vi "Actor Core.vi"(8 "error in":errorcluster, 11 "Nested in":refnum<class "Microscope Controller.lvclass">) -> (0 "error out":errorcluster, 3 "Actor out":refnum<class "Actor.lvclass">)   [LabVIEW 2020, in "Microscope.lvlib" / "Microscope Controller.lvlib" / "Microscope Controller.lvclass"]
doc: "(<B>Filename</B>: Actor Framework.lvlib:Actor.lvclass:Actor Core.vi)\n\nReceives messages to the actor, reacts to them, and initiates any error handling that may shut the actor down.\n\nDescendant classes may override this VI to append parallel tasks for the actor to complete while it handles messages. Overrides use the Call Parent Method node."
uses:
  Microscope Controller.lvclass
  C:/Program Files/National Instruments/LabVIEW 2020/vi.lib/ActorFramework/Actor/Actor.lvclass
  <vilib>/ActorFramework/Actor/Actor.lvclass
  <vilib>/ActorFramework/Actor/Actor.lvclass/Actor.ctl
  <vilib>/ActorFramework/Message Enqueuer/Message Enqueuer.lvclass/Message Enqueuer.ctl
  Microscope Controller.lvclass/Microscope Controller.ctl
  <vilib>/ActorFramework/Message Enqueuer/Init from Existing Queue.vi
  <vilib>/ActorFramework/Message Enqueuer/Enqueue.vi
  <vilib>/ActorFramework/Stop Msg/Stop Msg.lvclass
  C:/Program Files/National Instruments/LabVIEW 2020/vi.lib/ActorFramework/Message/Message.lvclass
  <vilib>/ActorFramework/Message Priority Queue/Priority Enqueue.vi
  <vilib>/ActorFramework/Message Enqueuer/Message Enqueuer.lvclass
panel:
  in  "Tab Control":T1(tab)
  out "SystemStatus":string
  # "430 Chemical and Biomedical Engineering Bldg.\nThe Pennsylvania State University"
  # "woh1@psu.edu"
  # "https://sites.psu.edu/hancocklab/"
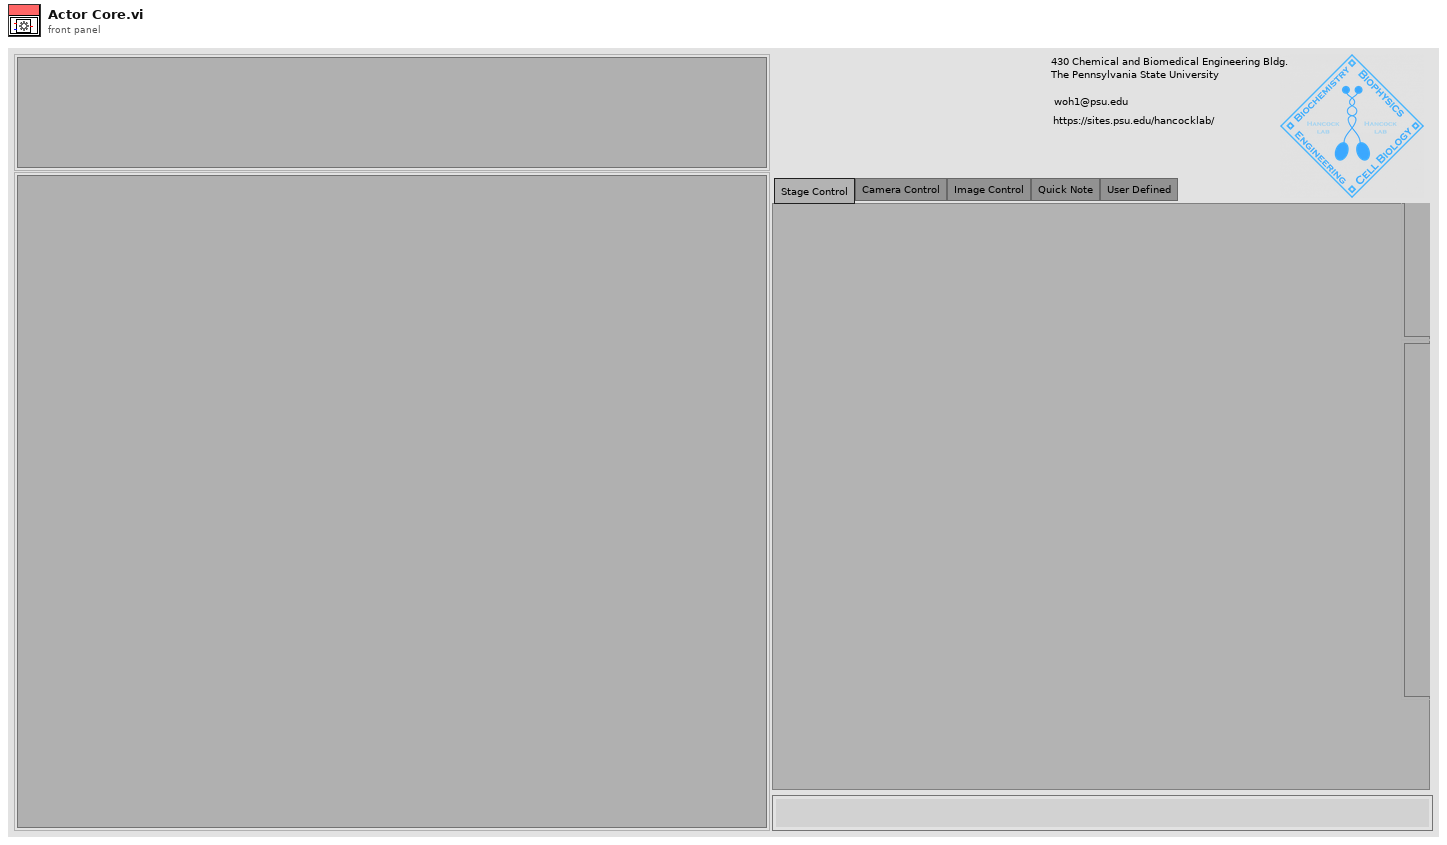
[diagram p1: front panel]
types:
  T1 = enum32{"Stage Control", "Camera Control", "Image Control", "Quick Note", "User Defined"}
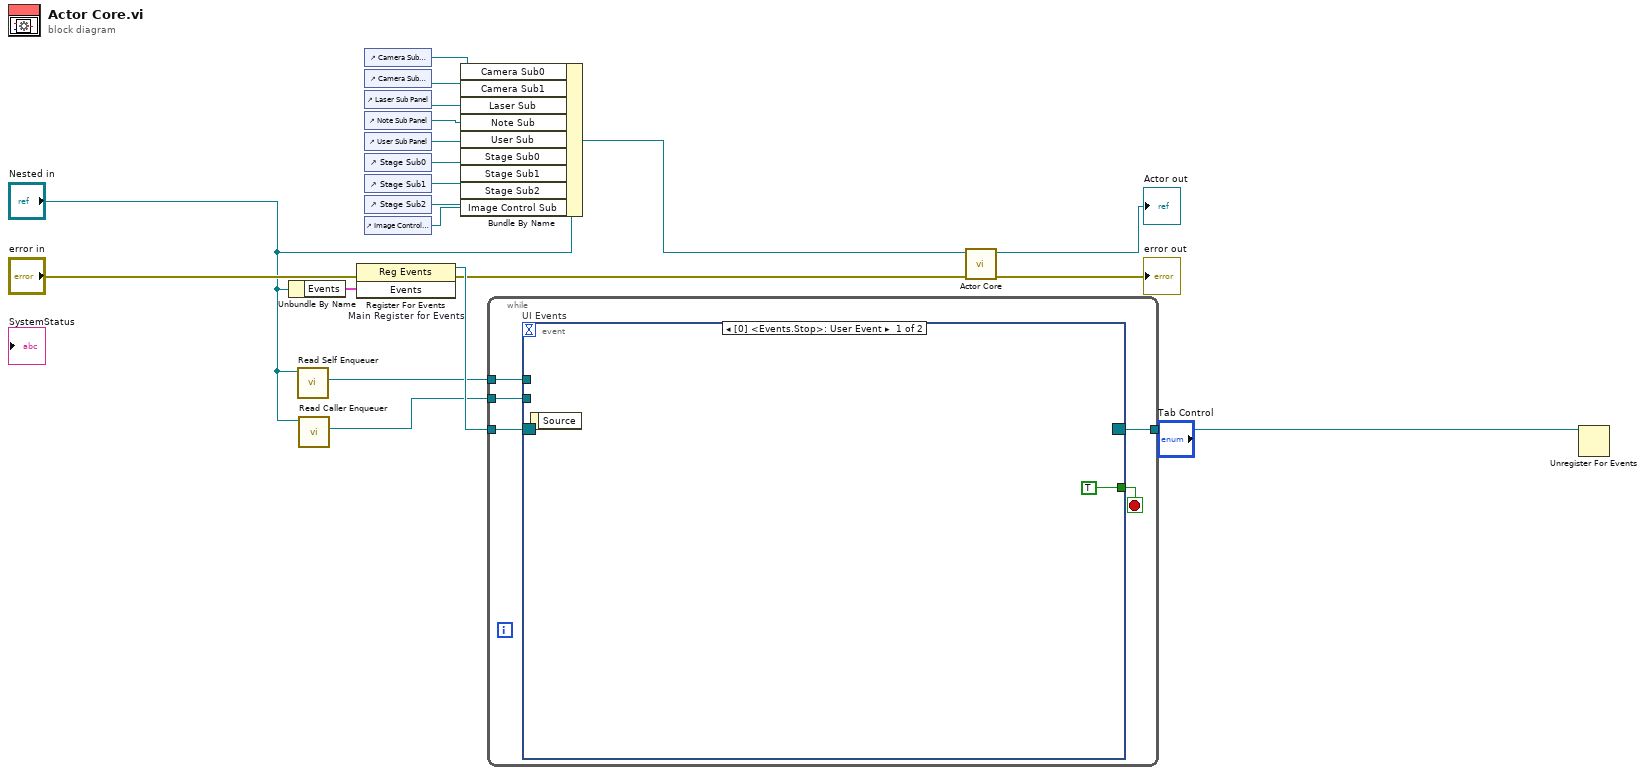
[diagram p0: block diagram]
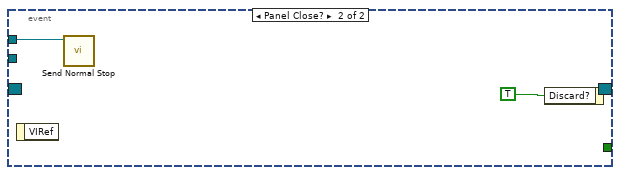
[diagram p2: hidden frame]
diagram:
  n1 = Unbundle By Name("Nested in") -> ("Events"=w17:cluster{"Stop":refnum<user-event>})
  n2 = call <vilib>:"Read Self Enqueuer.vi"("Actor"="Nested in") -> ("Self Enqueuer"=w15:refnum<class "Message Enqueuer.lvclass">)  [unwired: 10 in]
  n3 = call <vilib>:"Read Caller Enqueuer.vi"("Actor"="Nested in") -> ("Caller Enqueuer"=w12:refnum<class "Message Enqueuer.lvclass">)  [unwired: 10 in]
  n4 = register-events "Main Register for Events"(error in="error in", w17) -> (reference out=w18:refnum<event-registration>, error out=w13:errorcluster)  [unwired: 1 in]
  n5 = control-ref of="Camera Sub Panel0"() -> (w2:refnum<vi>)
  n6 = control-ref of="Camera Sub Panel1"() -> (w9:refnum<vi>)
  n7 = control-ref of="Laser Sub Panel"() -> (w8:refnum<vi>)
  n8 = control-ref of="Note Sub Panel"() -> (w7:refnum<vi>)
  n9 = control-ref of="User Sub Panel"() -> (w6:refnum<vi>)
  n10 = control-ref of="Stage Sub0"() -> (w3:refnum<vi>)
  n11 = control-ref of="Stage Sub1"() -> (w5:refnum<vi>)
  n12 = control-ref of="Stage Sub2"() -> (w4:refnum<vi>)
  n13 = control-ref of="Image Control Sub Panel"() -> (w1:refnum<vi>)
  n14 = Bundle By Name(cluster="Nested in", "Camera Sub0"=w2, "Camera Sub1"=w9, "Laser Sub"=w8, "Note Sub"=w7, "User Sub"=w6, "Stage Sub0"=w3, "Stage Sub1"=w5, "Stage Sub2"=w4, "Image Control Sub"=w1) -> (w10:refnum<class "Microscope Controller.lvclass">)
  n15 = while {
    tunnel: w18 -> [w25]
    tunnel: [w23] -> w16
    tunnel: w15 -> [w22]
    tunnel: w12 -> [w21]
    stop <- w24 stop-if-true
    n16 = event "UI Events" shown="[0] <Events.Stop>: User Event" {
      selector: w25 -> [_ _]
      dyn-events: [_ _] -> w23
      timeout: _ -> [_ _]
      tunnel: [TRUE _] -> w24
      tunnel: w22 -> [_ w27]
      tunnel: w21 -> [_ _]
      event User Event {
        n17 = event-data() -> ()  [unwired: 1 in, 1 out]
      }
      event Panel Close? {
        n18 = event-data() -> ()  [unwired: 1 in, 1 out]
        n19 = call <vilib>:"Send Normal Stop.vi"("Message Enqueuer"=w27) -> ()  [unwired: 10 in, 1 out]
        n20 = event-data("Discard?"=TRUE) -> ()  [unwired: 1 in, 1 out]
      }
    }
  }
  n21 = call-parent "Actor Core.vi"("error in"=w13, "Actor in"=w10) -> ("error out"=→"error out":errorcluster, "Actor out"=→"Actor out":refnum<class "Actor.lvclass">)  [unwired: 8 in]
  n22 = Unregister For Events(event registration refnum=w16) -> ()  [unwired: 1 in, 1 out]
